vi "Test Comm.vi"() -> ()   [LabVIEW 2021]
uses:
  CIFChannels/Typedef/Direction.ctl
  CIF_NIChn_Fifo_Power.lvclass
  ChannelCommon/typedef/FIFO Config.ctl
  ChannelCommon/typedef/Datatype Waveform.ctl
  CIFCore/Common/Utilities/Add Error.vi
  CIFCore/Common/Utilities/Append Error Location.vi
  ChannelCommon/ChannelCommon.lvlib
  CIFChannels/CIFChannels.lvclass
panel:
  out "status":string
  out "pass":bool
  out "error out":errorcluster
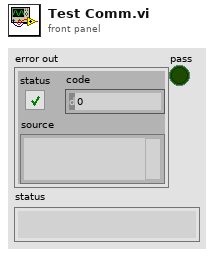
[diagram p1: front panel]
types:
  T1 = typedef "CIFChannels.lvclass/Direction.ctl" = enum16{"Publisher", "Subscriber"}
  T2 = typedef "ChannelCommon.lvlib/FIFO Config.ctl" = cluster{"Depth":u64, "Flags":u64}
  T3 = typedef "ChannelCommon.lvlib/Datatype Waveform.ctl" = cluster{"measurement":dbl[], "dT":dbl, "Timestamp":u64}
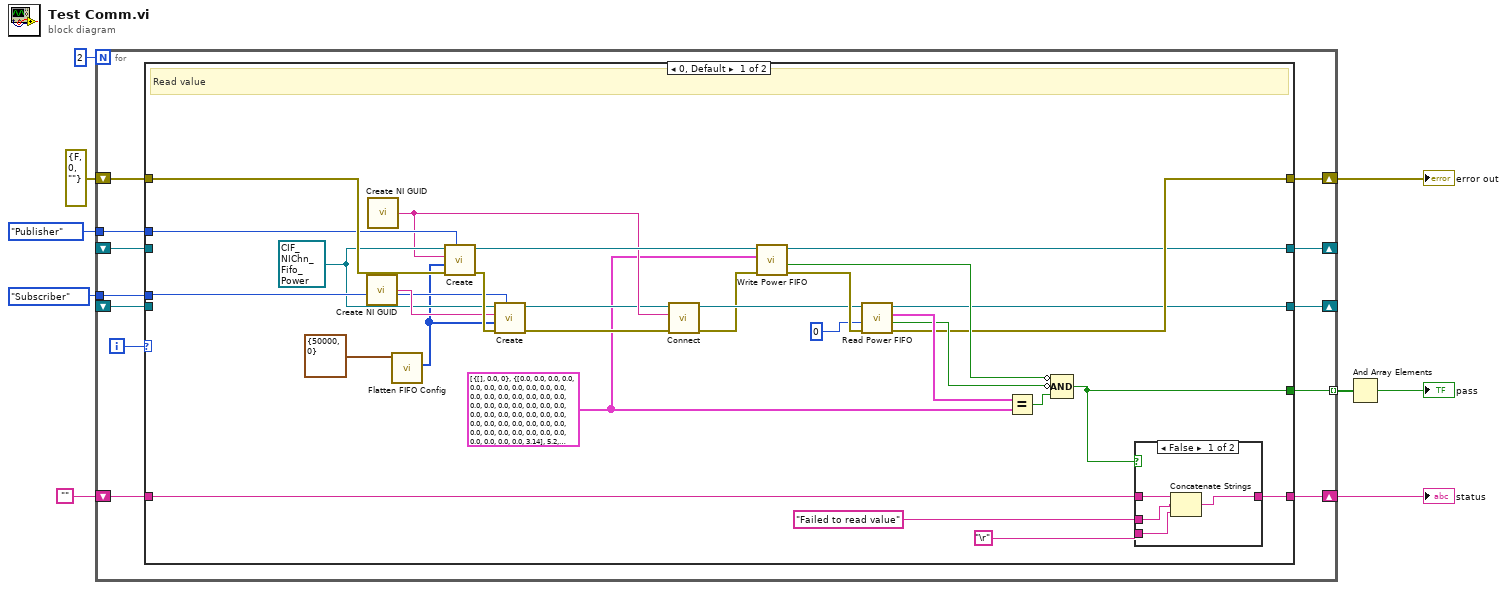
[diagram p0: block diagram]
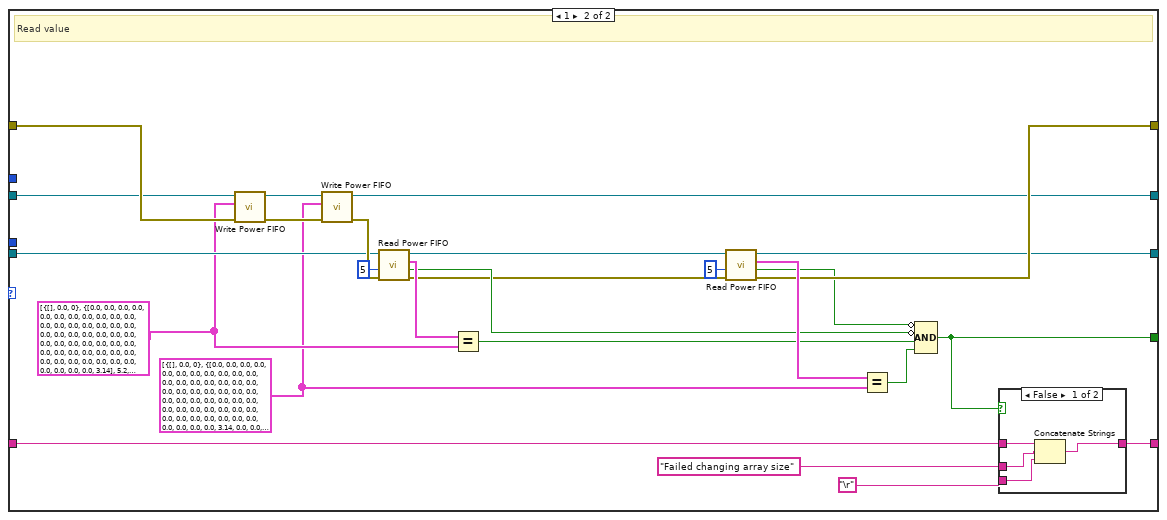
[diagram p3: hidden frame]
diagram:
  n1 = for {
    N: 2 -> [_]
    tunnel: [w21] -> w9 mode=indexing
    shift-right: [w19] -> w4
    shift-left: errorcluster {"status"=FALSE, "code"=0, "source"=""} ("error out") -> [w20]
    shift-right: [w16] -> w5
    shift-left: "" -> [w17]
    tunnel: Direction."Subscriber" ("Direction") -> [w15]
    tunnel: Direction."Publisher" ("Direction") -> [w14]
    shift-right: [w13] -> _
    shift-left: _ -> [w11]
    shift-right: [w12] -> _
    shift-left: _ -> [w10]
    i -> [w18]
    n2 = case shown="0, Default" w18 {
      tunnel: [w45 w76] -> w21
      tunnel: w20 -> [w43 w70]
      tunnel: [w26 w74] -> w19
      tunnel: w17 -> [w50 w80]
      tunnel: [w49 w79] -> w16
      tunnel: w15 -> [w41 _]
      tunnel: w14 -> [w40 _]
      tunnel: [w24 w73] -> w13
      tunnel: [w23 w72] -> w12
      tunnel: w10 -> [_ w56]
      tunnel: w11 -> [_ w59]
      frame 0, Default {
        w22 = T3[] [{"measurement"=[], "dT"=0.0, "Timestamp"=0}, {"measurement"=[0.0, 0.0, 0.0, 0.0, 0.0, 0.0, 0.0, 0.0, 0.0, 0.0, 0.0, 0.0, 0.0, 0.0, 0.0, 0.0, 0.0, 0.0, 0.0, 0.0, 0.0, 0.0, 0.0, 0.0, 0.0, 0.0, 0.0, 0.0, 0.0, 0.0, 0.0, 0.0, 0.0, 0.0, 0.0, 0.0, 0.0, 0.0, 0.0, 0.0, 0.0, 0.0, 0.0, 0.0, 0.0, 0.0, 0.0, 0.0, 0.0, 0.0, 3.14], "dT"=5.2, "Timestamp"=523}] ("Data In")
        w39 = refnum<class "CIF_NIChn_Fifo_Power.lvclass"> refnum ("CIF_NIChn_Fifo_Power.lvclass")
        # "Read value"
        n3 = call <vilib>:"Create NI GUID.vi"() -> ("NI GUID"=w42:string)
        n4 = call <vilib>:"Create NI GUID.vi"() -> ("NI GUID"=w30:string)
        n5 = call "Flatten FIFO Config.vi"("FIFO Config in"=T2 {"Depth"=50000, "Flags"=0}) -> ("Flattened Data out"=w37:u8[])  [unwired: 8 in, 2 out]
        n6 = call-dynamic "Create.vi"("Direction"=w40, "error in (no error)"=w43, "Custom Config Data"=w37, "Name"=w30, "CIFTag in"=w39) -> ("error out"=w44:errorcluster, "CIFTag out"=w36:refnum<class "CIF_NIChn_Fifo_Power.lvclass">)  [unwired: 5 in]
        n7 = call-dynamic "Create.vi"("Direction"=w41, "error in (no error)"=w44, "Custom Config Data"=w37, "Name"=w42, "CIFTag in"=w39) -> ("error out"=w29:errorcluster, "CIFTag out"=w27:refnum<class "CIF_NIChn_Fifo_Power.lvclass">)  [unwired: 5 in]
        n8 = call-dynamic "Connect.vi"("error in (no error)"=w29, "Connection Name"=w30, "CIFTag in"=w27) -> ("error out"=w28:errorcluster, "CIFTag out"=w31:refnum<class "CIF_NIChn_Fifo_Power.lvclass">)  [unwired: 7 in]
        n9 = call-dynamic "Write Power FIFO.vi"("error in (no error)"=w28, "Data In"=w22, "CIFTag in"=w36) -> ("error out"=w35:errorcluster, "timed out?"=w33:bool, "CIFTag out"=w23:refnum<class "CIF_NIChn_Fifo_Power.lvclass">)  [unwired: 5 in, 1 out]
        n10 = call-dynamic "Read Power FIFO.vi"("error in (no error)"=w35, "Timeout (ms)"=0, "CIFTag in"=w31) -> ("error out"=w26:errorcluster, "timed out?"=w32:bool, "Data out"=w34:T3[], "CIFTag out"=w24:refnum<class "CIF_NIChn_Fifo_Power.lvclass">)  [unwired: 4 in, 1 out]
        n11 = Equal?(x=w34, y=w22) -> (x = y?=w46:bool)
        n12 = Compound Arithmetic op=AND(invert w33, invert w32, w46) -> (w45:bool)
        n13 = case shown="False" w45 {
          tunnel: w50 -> [w54 w55]
          tunnel: [w51 w55] -> w49
          tunnel: "Failed to read value" -> [w53 _]
          tunnel: "\r" -> [w52 _]
          frame False {
            n14 = Concatenate Strings(w54, w53, w52) -> (w51:string)
          }
          frame True {
          }
        }
      }
      frame 1 {
        w57 = T3[] [{"measurement"=[], "dT"=0.0, "Timestamp"=0}, {"measurement"=[0.0, 0.0, 0.0, 0.0, 0.0, 0.0, 0.0, 0.0, 0.0, 0.0, 0.0, 0.0, 0.0, 0.0, 0.0, 0.0, 0.0, 0.0, 0.0, 0.0, 0.0, 0.0, 0.0, 0.0, 0.0, 0.0, 0.0, 0.0, 0.0, 0.0, 0.0, 0.0, 0.0, 0.0, 0.0, 0.0, 0.0, 0.0, 0.0, 0.0, 0.0, 0.0, 0.0, 0.0, 0.0, 0.0, 0.0, 0.0, 0.0, 0.0, 3.14, 0.0, 0.0, 0.0, 0.0, 0.0, 0.0, 0.0, 0.0, 0.0, 0.0, 0.0, 0.0, 0.0, 0.0, 0.0, 0.0, 0.0, 0.0, 0.0, 0.0, 0.0, 0.0, 0.0, 0.0, 0.0, 0.0, 0.0, 0.0, 0.0, 0.0, 0.0, 0.0, 0.0, 0.0, 0.0, 0.0, 0.0, 0.0, 0.0, 0.0, 0.0, 0.0, 0.0, 0.0, 0.0, 0.0, 0.0, 0.0, 0.0, 3.14], "dT"=5.2, "Timestamp"=523}] ("Data In")
        w58 = T3[] [{"measurement"=[], "dT"=0.0, "Timestamp"=0}, {"measurement"=[0.0, 0.0, 0.0, 0.0, 0.0, 0.0, 0.0, 0.0, 0.0, 0.0, 0.0, 0.0, 0.0, 0.0, 0.0, 0.0, 0.0, 0.0, 0.0, 0.0, 0.0, 0.0, 0.0, 0.0, 0.0, 0.0, 0.0, 0.0, 0.0, 0.0, 0.0, 0.0, 0.0, 0.0, 0.0, 0.0, 0.0, 0.0, 0.0, 0.0, 0.0, 0.0, 0.0, 0.0, 0.0, 0.0, 0.0, 0.0, 0.0, 0.0, 3.14], "dT"=5.2, "Timestamp"=523}] ("Data In")
        # "Read value"
        n15 = call-dynamic "Write Power FIFO.vi"("error in (no error)"=w70, "Data In"=w58, "CIFTag in"=w56) -> ("error out"=w64:errorcluster, "CIFTag out"=w71:refnum<class "CIF_NIChn_Fifo_Power.lvclass">)  [unwired: 5 in, 2 out]
        n16 = call-dynamic "Write Power FIFO.vi"("error in (no error)"=w64, "Data In"=w57, "CIFTag in"=w71) -> ("CIFTag out"=w72:refnum<class "CIF_NIChn_Fifo_Power.lvclass">)  [unwired: 5 in, 3 out]
        n17 = call-dynamic "Read Power FIFO.vi"("error in (no error)"=w64, "Timeout (ms)"=5, "CIFTag in"=w59) -> ("error out"=w63:errorcluster, "timed out?"=w65:bool, "Data out"=w69:T3[], "CIFTag out"=w62:refnum<class "CIF_NIChn_Fifo_Power.lvclass">)  [unwired: 4 in, 1 out]
        n18 = Equal?(x=w69, y=w58) -> (x = y?=w67:bool)
        n19 = call-dynamic "Read Power FIFO.vi"("error in (no error)"=w63, "Timeout (ms)"=5, "CIFTag in"=w62) -> ("error out"=w74:errorcluster, "timed out?"=w66:bool, "Data out"=w75:T3[], "CIFTag out"=w73:refnum<class "CIF_NIChn_Fifo_Power.lvclass">)  [unwired: 4 in, 1 out]
        n20 = Equal?(x=w75, y=w57) -> (x = y?=w68:bool)
        n21 = Compound Arithmetic op=AND(invert w66, invert w65, w67, w68) -> (w76:bool)
        n22 = case shown="False" w76 {
          tunnel: w80 -> [w84 w85]
          tunnel: [w81 w85] -> w79
          tunnel: "Failed changing array size" -> [w83 _]
          tunnel: "\r" -> [w82 _]
          frame False {
            n23 = Concatenate Strings(w84, w83, w82) -> (w81:string)
          }
          frame True {
          }
        }
      }
    }
  }
  "error out" <- w4
  "status" <- w5
  n24 = And Array Elements(Boolean array=w9) -> (logical AND=→"pass":bool)
